vi "vibration_ysn.vi"() -> ()   [LabVIEW 2015]
uses:
  <vilib>/measure/NI_MABase.lvlib
panel:
  in  "Cluster 1":T1={"frequency"=26, "frequency 2"=8, "frequency 3"=26, " frequency 4"=26}
  out "Numeric":i32
  in  "Cluster 0":T1={"frequency"=26, "frequency 2"=8, "frequency 3"=26, " frequency 4"=26}
  in  "y 2":i32
  in  "Boolean":bool
  out "Waveform Graph":waveform(dbl)[](graph)
  in  "y":i32
  in  "Cluster":T1
  in  "Set Button":bool
  in  "appended array":waveform(dbl)[](array[waveform])
  out "x-y":u32
  in  "amplitude":dbl=2.0 format="%0.2p"
  in  "amplitude 4":dbl=2.0 format="%0.2p"
  in  "amplitude 3":dbl=2.0 format="%0.2p"
  in  "amplitude 2":dbl=2.0 format="%0.2p"
  out "frequency 4":u32=20
  out "frequency 3":u32
  in  "sampling info 4":cluster{"Fs":dbl, "#s":dbl}={"Fs"=1000.0, "#s"=250.0} {"Fs" format="%.2p"}
  in  "sampling info 3":cluster{"Fs":dbl, "#s":dbl}={"Fs"=1000.0, "#s"=250.0} {"Fs" format="%.2p"}
  in  "signal type 4":T2(ring)
  in  "signal type 3":T2(ring)
  in  "signal type 2":T2(ring)
  in  "sampling info 2":cluster{"Fs":dbl, "#s":dbl}={"Fs"=1000.0, "#s"=250.0} {"Fs" format="%.2p"}
  out "frequency 2":u32=20
  out "frequency":u32=20
  in  "signal type":T2(ring)
  in  "sampling info":cluster{"Fs":dbl, "#s":dbl}={"Fs"=1000.0, "#s"=250.0} {"Fs" format="%.2p"}
  in  "stop (F)":bool
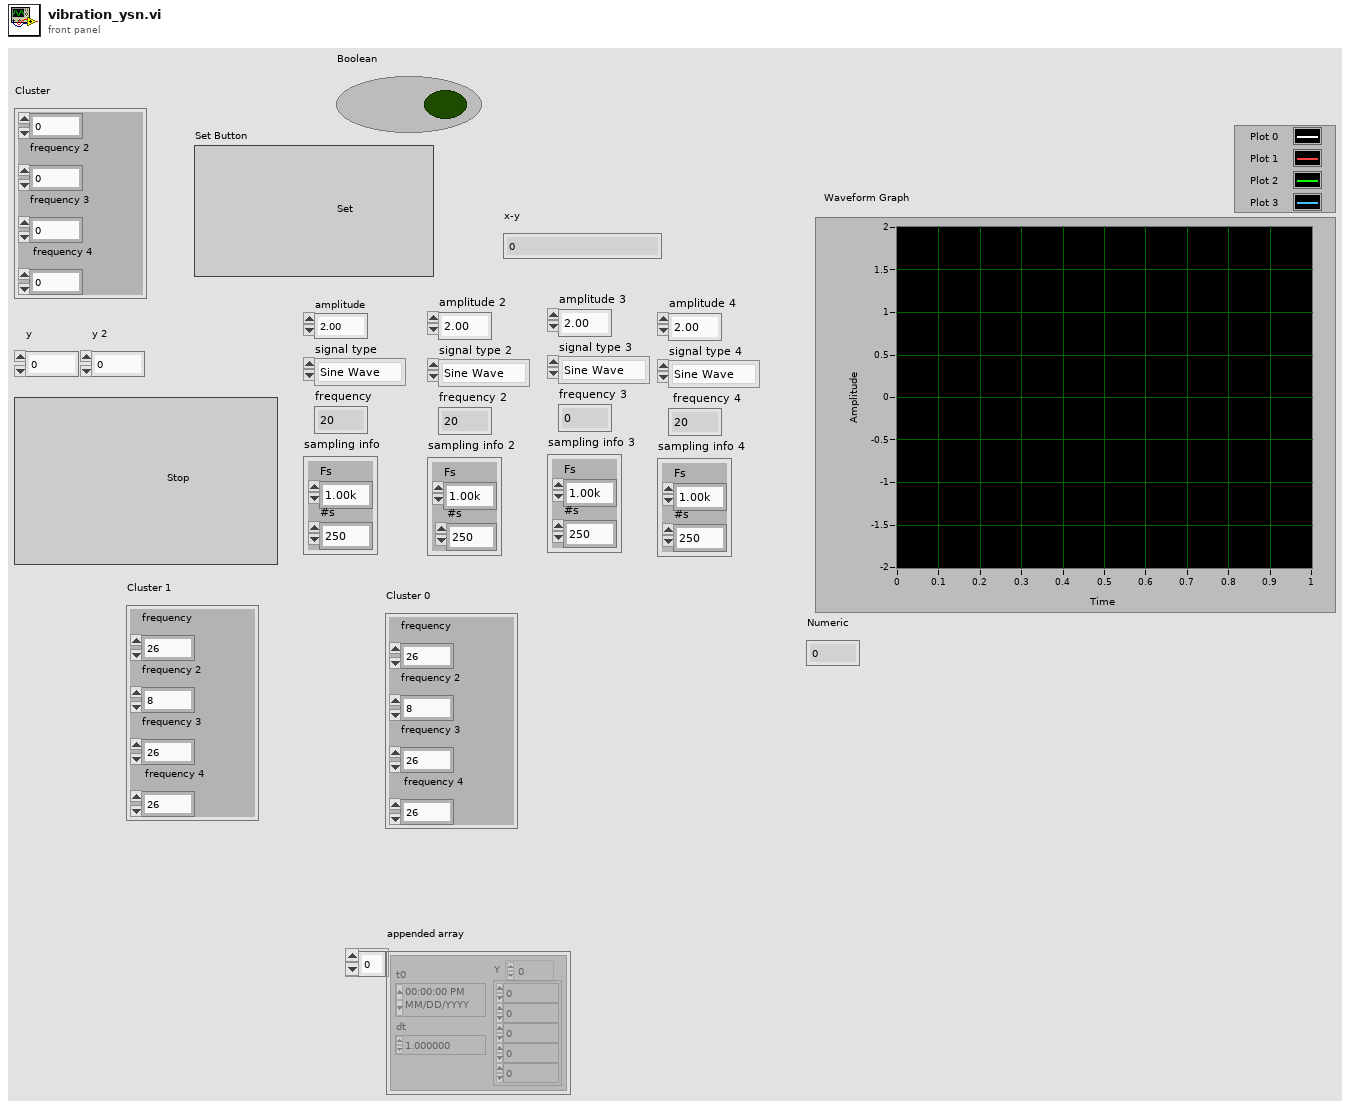
[diagram p1: front panel]
types:
  T1 = cluster{"frequency":u32, "frequency 2":u32, "frequency 3":u32, " frequency 4":u32}
  T2 = enum16{"Sine Wave", "Triangle Wave", "Square Wave", "Sawtooth Wave"}
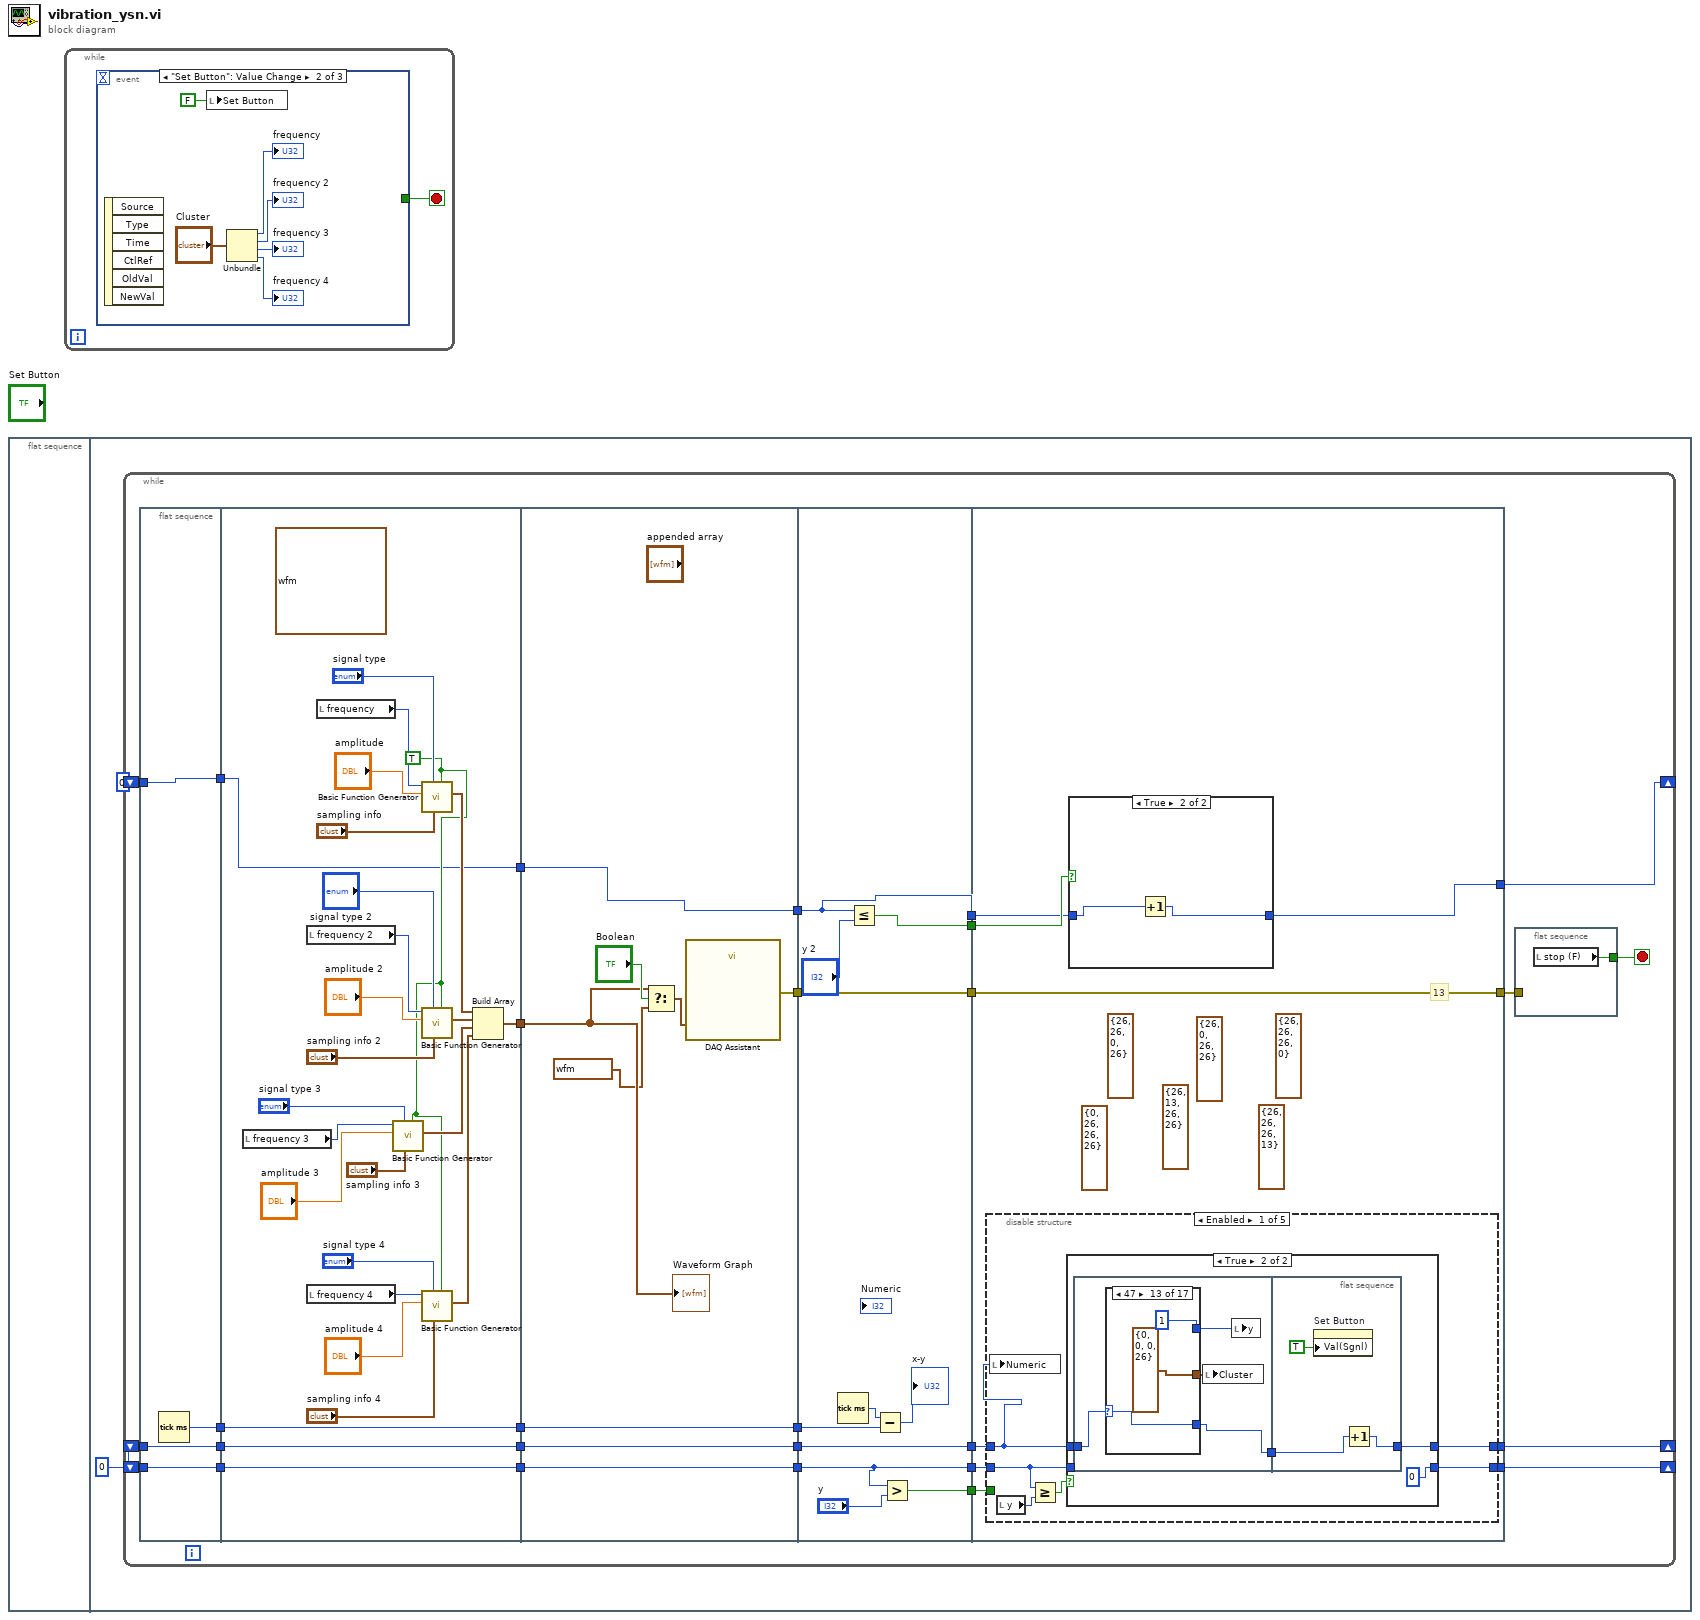
[diagram p0: block diagram]
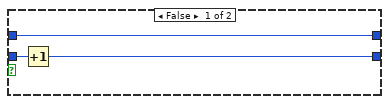
[diagram p2: hidden frame]
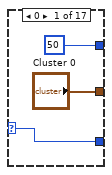
[diagram p3: hidden frame]
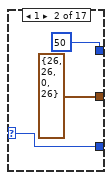
[diagram p4: hidden frame]
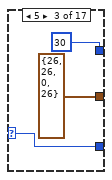
[diagram p5: hidden frame]
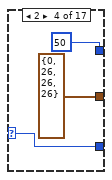
[diagram p6: hidden frame]
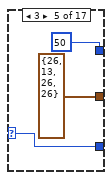
[diagram p7: hidden frame]
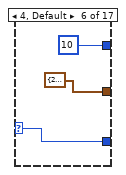
[diagram p8: hidden frame]
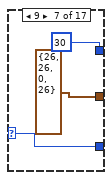
[diagram p9: hidden frame]
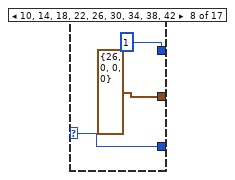
[diagram p10: hidden frame]
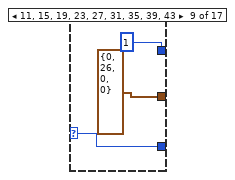
[diagram p11: hidden frame]
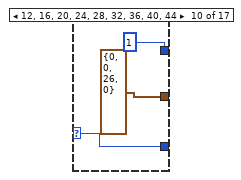
[diagram p12: hidden frame]
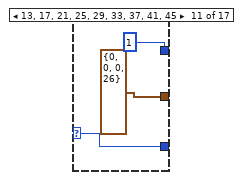
[diagram p13: hidden frame]
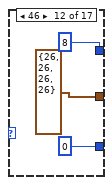
[diagram p14: hidden frame]
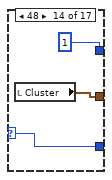
[diagram p15: hidden frame]
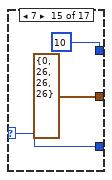
[diagram p16: hidden frame]
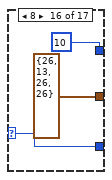
[diagram p17: hidden frame]
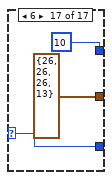
[diagram p18: hidden frame]
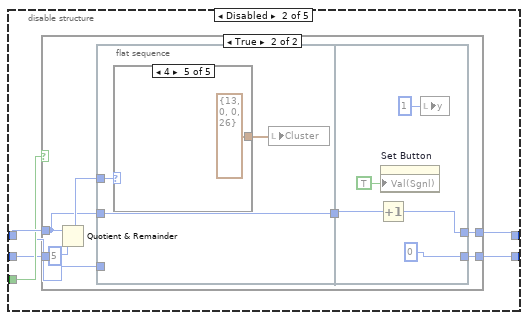
[diagram p19: hidden frame]
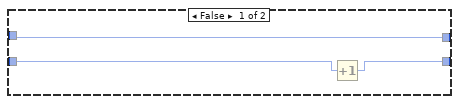
[diagram p20: hidden frame]
diagram:
  n1 = flat-sequence {
    frame #0 {
    }
    frame #1 {
      w2 = 0
      n2 = while {
        shift-right: [w19] -> _
        shift-left: w2 -> [w15]
        shift-right: [w11] -> _
        shift-left: w2 -> [w18]
        shift-right: [w6] -> _
        shift-left: 0 -> [w8]
        stop <- w30 stop-if-true
        n3 = flat-sequence {
          tunnel: [w34] -> w27
          tunnel: w18 -> [w33]
          tunnel: [w33] -> w17
          tunnel: w15 -> [w32]
          tunnel: [w32] -> w14
          tunnel: [w31] -> w9
          tunnel: w8 -> [w31]
          tunnel: [w45] -> w28
          tunnel: w27 -> [w45]
          tunnel: [w43] -> w24
          tunnel: [w37] -> w22
          tunnel: w17 -> [w38]
          tunnel: [w38] -> w16
          tunnel: w14 -> [w37]
          tunnel: [w35] -> w10
          tunnel: w9 -> [w35]
          tunnel: w28 -> [w69]
          tunnel: [w68] -> w26
          tunnel: [w69] -> w25
          tunnel: w24 -> [w63]
          tunnel: [w67] -> w23
          tunnel: w22 -> [w67]
          tunnel: w16 -> [w66]
          tunnel: [w66] -> w12
          tunnel: w10 -> [w65]
          tunnel: [w65] -> w7
          tunnel: w26 -> [w80]
          tunnel: w25 -> [w78]
          tunnel: w23 -> [w71]
          tunnel: [w80] -> w21
          tunnel: [w71] -> w20
          tunnel: [w76] -> w13
          tunnel: w12 -> [w76]
          tunnel: w7 -> [w74]
          tunnel: [w74] -> w5
          tunnel: [w73] -> w4
          tunnel: [w70] -> w3
          tunnel: [w89] -> w29
          tunnel: w21 -> [w89]
          tunnel: w20 -> [w87]
          tunnel: [w88] -> w19
          tunnel: w13 -> [w86]
          tunnel: [w85] -> w11
          tunnel: [w83] -> w6
          tunnel: w5 -> [w82]
          tunnel: w4 -> [w84]
          tunnel: w3 -> [w81]
          frame #0 {
            n4 = Tick Count (ms)() -> (millisecond timer value=w34:u32)
          }
          frame #1 {
            w36 = TRUE ("reset signal")
            (unwired) waveform(dbl) {"t0"=timestamp(0 s since 1904-01-01), "dt"=1.0, "Y"=[]} ("signal out")
            n5 = local read "frequency 3"() -> (w40:u32)
            n6 = local read "frequency 2"() -> (w41:u32)
            n7 = local read "frequency 4"() -> (w42:u32)
            n8 = local read "frequency"() -> (w39:u32)
            n9 = call <vilib>:"Basic Function Generator.vi"("reset signal"=w36, "sampling info"="sampling info 3", "signal type"="signal type 3", "amplitude"="amplitude 3", "frequency"=w40) -> ("signal out"=w51:waveform(dbl))  [unwired: 4 in, 2 out]
            n10 = call <vilib>:"Basic Function Generator.vi"("reset signal"=w36, "sampling info"="sampling info", "signal type"="signal type", "amplitude"="amplitude", "frequency"=w39) -> ("signal out"=w44:waveform(dbl))  [unwired: 4 in, 2 out]
            n11 = call <vilib>:"Basic Function Generator.vi"("reset signal"=w36, "sampling info"="sampling info 2", "signal type"="signal type 2", "amplitude"="amplitude 2", "frequency"=w41) -> ("signal out"=w57:waveform(dbl))  [unwired: 4 in, 2 out]
            n12 = call <vilib>:"Basic Function Generator.vi"("reset signal"=w36, "sampling info"="sampling info 4", "signal type"="signal type 4", "amplitude"="amplitude 4", "frequency"=w42) -> ("signal out"=w50:waveform(dbl))  [unwired: 4 in, 2 out]
            n13 = Build Array(w44, w57, w51, w50) -> (w43:waveform(dbl)[])
          }
          frame #2 {
            n14 = Select(t=w63, s="Boolean", f=waveform(dbl)[] [{"t0"=timestamp(0 s since 1904-01-01), "dt"=0.001, "Y"=[0.0, 0.0, 0.0, 0.0, 0.0, 0.0, 0.0, 0.0, 0.0, 0.0, 0.0, 0.0, 0.0, 0.0, 0.0, 0.0, 0.0, 0.0, 0.0, 0.0, 0.0, 0.0, 0.0, 0.0, 0.0, 0.0, 0.0, 0.0, 0.0, 0.0, 0.0, 0.0, 0.0, 0.0, 0.0, 0.0, 0.0, 0.0, 0.0, 0.0, 0.0, 0.0, 0.0, 0.0, 0.0, 0.0, 0.0, 0.0, 0.0, 0.0, 0.0, 0.0, 0.0, 0.0, 0.0, 0.0, 0.0, 0.0, 0.0, 0.0, 0.0, 0.0, 0.0, 0.0, 0.0, 0.0, 0.0, 0.0, 0.0, 0.0, 0.0, 0.0, 0.0, 0.0, 0.0, 0.0, 0.0, 0.0, 0.0, 0.0, 0.0, 0.0, 0.0, 0.0, 0.0, 0.0, 0.0, 0.0, 0.0, 0.0, 0.0, 0.0, 0.0, 0.0, 0.0, 0.0, 0.0, 0.0, 0.0, 0.0, 0.0, 0.0, 0.0, 0.0, 0.0, 0.0, 0.0, 0.0, 0.0, 0.0, 0.0, 0.0, 0.0, 0.0, 0.0, 0.0, 0.0, 0.0, 0.0, 0.0, 0.0, 0.0, 0.0, 0.0, 0.0, 0.0, 0.0, 0.0, 0.0, 0.0, 0.0, 0.0, 0.0, 0.0, 0.0, 0.0, 0.0, 0.0, 0.0, 0.0, 0.0, 0.0, 0.0, 0.0, 0.0, 0.0, 0.0, 0.0, 0.0, 0.0, 0.0, 0.0, 0.0, 0.0, 0.0, 0.0, 0.0, 0.0, 0.0, 0.0, 0.0, 0.0, 0.0, 0.0, 0.0, 0.0, 0.0, 0.0, 0.0, 0.0, 0.0, 0.0, 0.0, 0.0, 0.0, 0.0, 0.0, 0.0, 0.0, 0.0, 0.0, 0.0, 0.0, 0.0, 0.0, 0.0, 0.0, 0.0, 0.0, 0.0, 0.0, 0.0, 0.0, 0.0, 0.0, 0.0, 0.0, 0.0, 0.0, 0.0, 0.0, 0.0, 0.0, 0.0, 0.0, 0.0, 0.0, 0.0, 0.0, 0.0, 0.0, 0.0, 0.0, 0.0, 0.0, 0.0, 0.0, 0.0, 0.0, 0.0, 0.0, 0.0, 0.0, 0.0, 0.0, 0.0, 0.0, 0.0, 0.0, 0.0, 0.0, 0.0, 0.0, 0.0, 0.0, 0.0, 0.0, 0.0, 0.0, 0.0, 0.0, 0.0, 0.0, 0.0, 0.0, 0.0, 0.0, 0.0, 0.0, 0.0]}, {"t0"=timestamp(0 s since 1904-01-01), "dt"=0.001, "Y"=[0.0, 0.0, 0.0, 0.0, 0.0, 0.0, 0.0, 0.0, 0.0, 0.0, 0.0, 0.0, 0.0, 0.0, 0.0, 0.0, 0.0, 0.0, 0.0, 0.0, 0.0, 0.0, 0.0, 0.0, 0.0, 0.0, 0.0, 0.0, 0.0, 0.0, 0.0, 0.0, 0.0, 0.0, 0.0, 0.0, 0.0, 0.0, 0.0, 0.0, 0.0, 0.0, 0.0, 0.0, 0.0, 0.0, 0.0, 0.0, 0.0, 0.0, 0.0, 0.0, 0.0, 0.0, 0.0, 0.0, 0.0, 0.0, 0.0, 0.0, 0.0, 0.0, 0.0, 0.0, 0.0, 0.0, 0.0, 0.0, 0.0, 0.0, 0.0, 0.0, 0.0, 0.0, 0.0, 0.0, 0.0, 0.0, 0.0, 0.0, 0.0, 0.0, 0.0, 0.0, 0.0, 0.0, 0.0, 0.0, 0.0, 0.0, 0.0, 0.0, 0.0, 0.0, 0.0, 0.0, 0.0, 0.0, 0.0, 0.0, 0.0, 0.0, 0.0, 0.0, 0.0, 0.0, 0.0, 0.0, 0.0, 0.0, 0.0, 0.0, 0.0, 0.0, 0.0, 0.0, 0.0, 0.0, 0.0, 0.0, 0.0, 0.0, 0.0, 0.0, 0.0, 0.0, 0.0, 0.0, 0.0, 0.0, 0.0, 0.0, 0.0, 0.0, 0.0, 0.0, 0.0, 0.0, 0.0, 0.0, 0.0, 0.0, 0.0, 0.0, 0.0, 0.0, 0.0, 0.0, 0.0, 0.0, 0.0, 0.0, 0.0, 0.0, 0.0, 0.0, 0.0, 0.0, 0.0, 0.0, 0.0, 0.0, 0.0, 0.0, 0.0, 0.0, 0.0, 0.0, 0.0, 0.0, 0.0, 0.0, 0.0, 0.0, 0.0, 0.0, 0.0, 0.0, 0.0, 0.0, 0.0, 0.0, 0.0, 0.0, 0.0, 0.0, 0.0, 0.0, 0.0, 0.0, 0.0, 0.0, 0.0, 0.0, 0.0, 0.0, 0.0, 0.0, 0.0, 0.0, 0.0, 0.0, 0.0, 0.0, 0.0, 0.0, 0.0, 0.0, 0.0, 0.0, 0.0, 0.0, 0.0, 0.0, 0.0, 0.0, 0.0, 0.0, 0.0, 0.0, 0.0, 0.0, 0.0, 0.0, 0.0, 0.0, 0.0, 0.0, 0.0, 0.0, 0.0, 0.0, 0.0, 0.0, 0.0, 0.0, 0.0, 0.0, 0.0, 0.0, 0.0, 0.0, 0.0, 0.0, 0.0, 0.0, 0.0, 0.0, 0.0, 0.0]}, {"t0"=timestamp(0 s since 1904-01-01), "dt"=0.001, "Y"=[0.0, 0.0, 0.0, 0.0, 0.0, 0.0, 0.0, 0.0, 0.0, 0.0, 0.0, 0.0, 0.0, 0.0, 0.0, 0.0, 0.0, 0.0, 0.0, 0.0, 0.0, 0.0, 0.0, 0.0, 0.0, 0.0, 0.0, 0.0, 0.0, 0.0, 0.0, 0.0, 0.0, 0.0, 0.0, 0.0, 0.0, 0.0, 0.0, 0.0, 0.0, 0.0, 0.0, 0.0, 0.0, 0.0, 0.0, 0.0, 0.0, 0.0, 0.0, 0.0, 0.0, 0.0, 0.0, 0.0, 0.0, 0.0, 0.0, 0.0, 0.0, 0.0, 0.0, 0.0, 0.0, 0.0, 0.0, 0.0, 0.0, 0.0, 0.0, 0.0, 0.0, 0.0, 0.0, 0.0, 0.0, 0.0, 0.0, 0.0, 0.0, 0.0, 0.0, 0.0, 0.0, 0.0, 0.0, 0.0, 0.0, 0.0, 0.0, 0.0, 0.0, 0.0, 0.0, 0.0, 0.0, 0.0, 0.0, 0.0, 0.0, 0.0, 0.0, 0.0, 0.0, 0.0, 0.0, 0.0, 0.0, 0.0, 0.0, 0.0, 0.0, 0.0, 0.0, 0.0, 0.0, 0.0, 0.0, 0.0, 0.0, 0.0, 0.0, 0.0, 0.0, 0.0, 0.0, 0.0, 0.0, 0.0, 0.0, 0.0, 0.0, 0.0, 0.0, 0.0, 0.0, 0.0, 0.0, 0.0, 0.0, 0.0, 0.0, 0.0, 0.0, 0.0, 0.0, 0.0, 0.0, 0.0, 0.0, 0.0, 0.0, 0.0, 0.0, 0.0, 0.0, 0.0, 0.0, 0.0, 0.0, 0.0, 0.0, 0.0, 0.0, 0.0, 0.0, 0.0, 0.0, 0.0, 0.0, 0.0, 0.0, 0.0, 0.0, 0.0, 0.0, 0.0, 0.0, 0.0, 0.0, 0.0, 0.0, 0.0, 0.0, 0.0, 0.0, 0.0, 0.0, 0.0, 0.0, 0.0, 0.0, 0.0, 0.0, 0.0, 0.0, 0.0, 0.0, 0.0, 0.0, 0.0, 0.0, 0.0, 0.0, 0.0, 0.0, 0.0, 0.0, 0.0, 0.0, 0.0, 0.0, 0.0, 0.0, 0.0, 0.0, 0.0, 0.0, 0.0, 0.0, 0.0, 0.0, 0.0, 0.0, 0.0, 0.0, 0.0, 0.0, 0.0, 0.0, 0.0, 0.0, 0.0, 0.0, 0.0, 0.0, 0.0, 0.0, 0.0, 0.0, 0.0, 0.0, 0.0, 0.0, 0.0, 0.0, 0.0, 0.0, 0.0]}, {"t0"=timestamp(0 s since 1904-01-01), "dt"=0.001, "Y"=[0.0, 0.0, 0.0, 0.0, 0.0, 0.0, 0.0, 0.0, 0.0, 0.0, 0.0, 0.0, 0.0, 0.0, 0.0, 0.0, 0.0, 0.0, 0.0, 0.0, 0.0, 0.0, 0.0, 0.0, 0.0, 0.0, 0.0, 0.0, 0.0, 0.0, 0.0, 0.0, 0.0, 0.0, 0.0, 0.0, 0.0, 0.0, 0.0, 0.0, 0.0, 0.0, 0.0, 0.0, 0.0, 0.0, 0.0, 0.0, 0.0, 0.0, 0.0, 0.0, 0.0, 0.0, 0.0, 0.0, 0.0, 0.0, 0.0, 0.0, 0.0, 0.0, 0.0, 0.0, 0.0, 0.0, 0.0, 0.0, 0.0, 0.0, 0.0, 0.0, 0.0, 0.0, 0.0, 0.0, 0.0, 0.0, 0.0, 0.0, 0.0, 0.0, 0.0, 0.0, 0.0, 0.0, 0.0, 0.0, 0.0, 0.0, 0.0, 0.0, 0.0, 0.0, 0.0, 0.0, 0.0, 0.0, 0.0, 0.0, 0.0, 0.0, 0.0, 0.0, 0.0, 0.0, 0.0, 0.0, 0.0, 0.0, 0.0, 0.0, 0.0, 0.0, 0.0, 0.0, 0.0, 0.0, 0.0, 0.0, 0.0, 0.0, 0.0, 0.0, 0.0, 0.0, 0.0, 0.0, 0.0, 0.0, 0.0, 0.0, 0.0, 0.0, 0.0, 0.0, 0.0, 0.0, 0.0, 0.0, 0.0, 0.0, 0.0, 0.0, 0.0, 0.0, 0.0, 0.0, 0.0, 0.0, 0.0, 0.0, 0.0, 0.0, 0.0, 0.0, 0.0, 0.0, 0.0, 0.0, 0.0, 0.0, 0.0, 0.0, 0.0, 0.0, 0.0, 0.0, 0.0, 0.0, 0.0, 0.0, 0.0, 0.0, 0.0, 0.0, 0.0, 0.0, 0.0, 0.0, 0.0, 0.0, 0.0, 0.0, 0.0, 0.0, 0.0, 0.0, 0.0, 0.0, 0.0, 0.0, 0.0, 0.0, 0.0, 0.0, 0.0, 0.0, 0.0, 0.0, 0.0, 0.0, 0.0, 0.0, 0.0, 0.0, 0.0, 0.0, 0.0, 0.0, 0.0, 0.0, 0.0, 0.0, 0.0, 0.0, 0.0, 0.0, 0.0, 0.0, 0.0, 0.0, 0.0, 0.0, 0.0, 0.0, 0.0, 0.0, 0.0, 0.0, 0.0, 0.0, 0.0, 0.0, 0.0, 0.0, 0.0, 0.0, 0.0, 0.0, 0.0, 0.0, 0.0, 0.0, 0.0, 0.0, 0.0, 0.0, 0.0, 0.0]}]) -> (s? t:f=w62:waveform(dbl)[])
            n15 = call "DAQ Assistant"("data"=w62) -> ("error out"=w68:errorcluster)  [unwired: 17 in, 1 out]
            "Waveform Graph" <- w63
          }
          frame #3 {
            n16 = Tick Count (ms)() -> (millisecond timer value=w79:u32)
            n17 = Less Or Equal?(x=w74, y="y 2") -> (x <= y?=w73:bool)
            n18 = Subtract(x=w79, y=w78) -> (x-y=→"x-y":u32)
            n19 = Greater?(x=w71, y="y") -> (0:w70:bool)
          }
          frame #4 {
            (unwired) T1 {"frequency"=26, "frequency 2"=26, "frequency 3"=26, " frequency 4"=13} ("Cluster 8")
            (unwired) T1 {"frequency"=26, "frequency 2"=13, "frequency 3"=26, " frequency 4"=26} ("Cluster 7")
            (unwired) T1 {"frequency"=0, "frequency 2"=26, "frequency 3"=26, " frequency 4"=26} ("Cluster 6")
            (unwired) T1 {"frequency"=26, "frequency 2"=26, "frequency 3"=26, " frequency 4"=0} ("Cluster")
            (unwired) T1 {"frequency"=26, "frequency 2"=0, "frequency 3"=26, " frequency 4"=26} ("Cluster")
            (unwired) T1 {"frequency"=26, "frequency 2"=26, "frequency 3"=0, " frequency 4"=26} ("Cluster")
            # "13"
            n20 = disable-structure shown="Enabled" {
              disable-tunnel: [w95 w163 _ w193 w261] -> w88
              disable-tunnel: w87 -> [w94 w161 _ w192 w260]
              disable-tunnel: w86 -> [w91 w165 _ w189 w256]
              disable-tunnel: [w93 w164 _ w191 w259] -> w85
              disable-tunnel: w81 -> [_ w162 _ _ _]
              frame Enabled {
                n21 = local write "Numeric"(w91) -> ()
                n22 = local read "y"() -> (w90:i32)
                n23 = Greater Or Equal?(x=w94, y=w90) -> (x >= y?=w92:bool)
                n24 = case shown="True" w92 {
                  tunnel: [w97 0] -> w95
                  tunnel: w94 -> [w98 _]
                  tunnel: w91 -> [w96 w101]
                  tunnel: [w96 w100] -> w93
                  frame False {
                    n25 = Increment(x=w98) -> (x+1=w97:i32)
                  }
                  frame True {
                    n26 = flat-sequence {
                      tunnel: w101 -> [w103]
                      tunnel: [w105] -> w99
                      tunnel: [w160] -> w100
                      tunnel: w99 -> [w159]
                      frame #0 {
                        n27 = case shown="47" w103 {
                          selector: w103 -> [w108 w111 w114 w117 w120 w123 w125 w128 w131 w134 w137 _ w143 w147 w150 w153 w155]
                          tunnel: ["Cluster 0" T1 {"frequency"=26, "frequency 2"=26, "frequency 3"=0, " frequency 4"=26} ("Cluster 1") T1 {"frequency"=26, "frequency 2"=26, "frequency 3"=0, " frequency 4"=26} ("Cluster 1") T1 {"frequency"=0, "frequency 2"=26, "frequency 3"=26, " frequency 4"=26} ("Cluster 2") T1 {"frequency"=26, "frequency 2"=13, "frequency 3"=26, " frequency 4"=26} ("Cluster 3") T1 {"frequency"=26, "frequency 2"=26, "frequency 3"=26, " frequency 4"=13} ("Cluster 4") T1 {"frequency"=26, "frequency 2"=26, "frequency 3"=0, " frequency 4"=26} ("Cluster 5") T1 {"frequency"=26, "frequency 2"=0, "frequency 3"=0, " frequency 4"=0} ("Cluster 5") T1 {"frequency"=0, "frequency 2"=26, "frequency 3"=0, " frequency 4"=0} ("Cluster 5") T1 {"frequency"=0, "frequency 2"=0, "frequency 3"=26, " frequency 4"=0} ("Cluster 5") T1 {"frequency"=0, "frequency 2"=0, "frequency 3"=0, " frequency 4"=26} ("Cluster 5") T1 {"frequency"=26, "frequency 2"=26, "frequency 3"=26, " frequency 4"=26} ("Cluster 5") T1 {"frequency"=0, "frequency 2"=0, "frequency 3"=0, " frequency 4"=26} ("Cluster 5") w146 T1 {"frequency"=0, "frequency 2"=26, "frequency 3"=26, " frequency 4"=26} ("Cluster 6") T1 {"frequency"=26, "frequency 2"=13, "frequency 3"=26, " frequency 4"=26} ("Cluster 6") T1 {"frequency"=26, "frequency 2"=26, "frequency 3"=26, " frequency 4"=13} ("Cluster 6")] -> w106
                          tunnel: [w108 w111 w114 w117 w120 w123 w125 w128 w131 w134 w137 0 w143 w147 w150 w153 w155] -> w105
                          tunnel: [50 ("y") 50 ("y") 30 ("y") 50 ("y") 50 ("y") 10 ("y") 30 ("y") 1 ("y") 1 ("y") 1 ("y") 1 ("y") 8 ("y") 1 ("y") 1 ("y") 10 ("y") 10 ("y") 10 ("y")] -> w104
                          frame 0 {
                          }
                          frame 1 {
                          }
                          frame 5 {
                          }
                          frame 2 {
                          }
                          frame 3 {
                          }
                          frame 4, Default {
                          }
                          frame 9 {
                          }
                          frame 10, 14, 18, 22, 26, 30, 34, 38, 42 {
                          }
                          frame 11, 15, 19, 23, 27, 31, 35, 39, 43 {
                          }
                          frame 12, 16, 20, 24, 28, 32, 36, 40, 44 {
                          }
                          frame 13, 17, 21, 25, 29, 33, 37, 41, 45 {
                          }
                          frame 46 {
                          }
                          frame 47 {
                          }
                          frame 48 {
                            n28 = local read "Cluster"() -> (w146:T1)
                          }
                          frame 7 {
                          }
                          frame 8 {
                          }
                          frame 6 {
                          }
                        }
                        n29 = local write "Cluster"(w106) -> ()
                        n30 = local write "y"(w104) -> ()
                      }
                      frame #1 {
                        n31 = property on="Set Button" class="Bool (strict)"("Val(Sgnl)"=TRUE ("Value (Signaling)")) -> ()  [unwired: 2 in, 2 out]
                        n32 = Increment(x=w159) -> (x+1=w160:i32)
                      }
                    }
                  }
                }
              }
              frame Disabled {
                n33 = case shown="True" w162 {
                  tunnel: w165 -> [w166 w169]
                  tunnel: [w166 w172] -> w164
                  tunnel: [w167 w171] -> w163
                  tunnel: w161 -> [w168 _]
                  frame False {
                    n34 = Increment(x=w168) -> (x+1=w167:i32)
                  }
                  frame True {
                    n35 = Quotient & Remainder(x=w169, y=5) -> (x-y*floor(x/y)=w173:i32)  [unwired: 1 out]
                    n36 = flat-sequence {
                      tunnel: w173 -> [w177]
                      tunnel: w169 -> [_]
                      tunnel: [w175] -> w170
                      tunnel: w169 -> [w175]
                      tunnel: [w184] -> w172
                      tunnel: [0] -> w171
                      tunnel: w170 -> [w185]
                      frame #0 {
                        n37 = case shown="4" w177 {
                          tunnel: [T1 {"frequency"=26, "frequency 2"=26, "frequency 3"=26, " frequency 4"=26} ("Cluster 6") T1 {"frequency"=26, "frequency 2"=13, "frequency 3"=0, " frequency 4"=0} ("Cluster 6") T1 {"frequency"=0, "frequency 2"=26, "frequency 3"=13, " frequency 4"=0} ("Cluster 6") T1 {"frequency"=0, "frequency 2"=0, "frequency 3"=26, " frequency 4"=13} ("Cluster 6") T1 {"frequency"=13, "frequency 2"=0, "frequency 3"=0, " frequency 4"=26} ("Cluster 6")] -> w176
                          frame 0, Default {
                          }
                          frame 1 {
                          }
                          frame 3 {
                          }
                          frame 2 {
                          }
                          frame 4 {
                          }
                        }
                        n38 = local write "Cluster"(w176) -> ()
                      }
                      frame #1 {
                        n39 = Increment(x=w185) -> (x+1=w184:i32)
                        n40 = property on="Set Button" class="Bool (strict)"("Val(Sgnl)"=TRUE ("Value (Signaling)")) -> ()  [unwired: 2 in, 2 out]
                        n41 = local write "y"(1 ("y")) -> ()
                      }
                    }
                  }
                }
              }
              frame Disabled {
              }
              frame Disabled {
                n42 = local write "Numeric"(w189) -> ()
                n43 = local read "y"() -> (w188:i32)
                n44 = Greater Or Equal?(x=w192, y=w188) -> (x >= y?=w190:bool)
                n45 = case shown="True" w190 {
                  tunnel: [w195 0] -> w193
                  tunnel: w192 -> [w196 _]
                  tunnel: w189 -> [w194 w199]
                  tunnel: [w194 w198] -> w191
                  frame False {
                    n46 = Increment(x=w196) -> (x+1=w195:i32)
                  }
                  frame True {
                    n47 = flat-sequence {
                      tunnel: w199 -> [w203]
                      tunnel: [w202] -> w197
                      tunnel: [w254] -> w198
                      tunnel: w197 -> [w253]
                      frame #0 {
                        n48 = case shown="10, 14, 18, 22, 26, 30, 34, 38, 42" w203 {
                          selector: w203 -> [w206 w209 w212 w215 w218 w221 w223 w226 w229 w232 w235 _ w241 w245 w248 w250]
                          tunnel: ["Cluster 1" T1 {"frequency"=26, "frequency 2"=26, "frequency 3"=0, " frequency 4"=26} ("Cluster 1") T1 {"frequency"=26, "frequency 2"=26, "frequency 3"=0, " frequency 4"=26} ("Cluster 1") T1 {"frequency"=0, "frequency 2"=26, "frequency 3"=26, " frequency 4"=26} ("Cluster 2") T1 {"frequency"=26, "frequency 2"=13, "frequency 3"=26, " frequency 4"=26} ("Cluster 3") T1 {"frequency"=26, "frequency 2"=26, "frequency 3"=26, " frequency 4"=13} ("Cluster 4") T1 {"frequency"=26, "frequency 2"=26, "frequency 3"=0, " frequency 4"=26} ("Cluster 5") T1 {"frequency"=26, "frequency 2"=0, "frequency 3"=0, " frequency 4"=0} ("Cluster 5") T1 {"frequency"=0, "frequency 2"=26, "frequency 3"=0, " frequency 4"=0} ("Cluster 5") T1 {"frequency"=0, "frequency 2"=0, "frequency 3"=26, " frequency 4"=0} ("Cluster 5") T1 {"frequency"=0, "frequency 2"=0, "frequency 3"=0, " frequency 4"=26} ("Cluster 5") T1 {"frequency"=26, "frequency 2"=26, "frequency 3"=26, " frequency 4"=26} ("Cluster 5") T1 {"frequency"=0, "frequency 2"=0, "frequency 3"=0, " frequency 4"=26} ("Cluster 5") T1 {"frequency"=0, "frequency 2"=26, "frequency 3"=26, " frequency 4"=26} ("Cluster 6") T1 {"frequency"=26, "frequency 2"=13, "frequency 3"=26, " frequency 4"=26} ("Cluster 6") T1 {"frequency"=26, "frequency 2"=26, "frequency 3"=26, " frequency 4"=13} ("Cluster 6")] -> w204
                          tunnel: [w206 w209 w212 w215 w218 w221 w223 w226 w229 w232 w235 0 w241 w245 w248 w250] -> w202
                          tunnel: [50 ("y") 50 ("y") 30 ("y") 50 ("y") 50 ("y") 10 ("y") 30 ("y") 1 ("y") 1 ("y") 1 ("y") 1 ("y") 8 ("y") 1 ("y") 10 ("y") 10 ("y") 10 ("y")] -> w201
                          frame 0 {
                          }
                          frame 1 {
                          }
                          frame 5 {
                          }
                          frame 2 {
                          }
                          frame 3 {
                          }
                          frame 4, Default {
                          }
                          frame 9 {
                          }
                          frame 10, 14, 18, 22, 26, 30, 34, 38, 42 {
                          }
                          frame 11, 15, 19, 23, 27, 31, 35, 39, 43 {
                          }
                          frame 12, 16, 20, 24, 28, 32, 36, 40, 44 {
                          }
                          frame 13, 17, 21, 25, 29, 33, 37, 41, 45 {
                          }
                          frame 46 {
                          }
                          frame 47 {
                          }
                          frame 7 {
                          }
                          frame 8 {
                          }
                          frame 6 {
                          }
                        }
                        n49 = local write "Cluster"(w204) -> ()
                        n50 = local write "y"(w201) -> ()
                      }
                      frame #1 {
                        n51 = property on="Set Button" class="Bool (strict)"("Val(Sgnl)"=TRUE ("Value (Signaling)")) -> ()  [unwired: 2 in, 2 out]
                        n52 = Increment(x=w253) -> (x+1=w254:i32)
                      }
                    }
                  }
                }
              }
              frame Disabled {
                n53 = local read "y"() -> (w257:i32)
                n54 = local write "Numeric"(w256) -> ()
                n55 = Greater Or Equal?(x=w260, y=w257) -> (x >= y?=w258:bool)
                n56 = case shown="True" w258 {
                  tunnel: [w263 0] -> w261
                  tunnel: w260 -> [w264 _]
                  tunnel: w256 -> [w262 w267]
                  tunnel: [w262 w266] -> w259
                  frame False {
                    n57 = Increment(x=w264) -> (x+1=w263:i32)
                  }
                  frame True {
                    n58 = flat-sequence {
                      tunnel: w267 -> [w271]
                      tunnel: [w270] -> w265
                      tunnel: [w304] -> w266
                      tunnel: w265 -> [w303]
                      frame #0 {
                        n59 = case shown="0" w271 {
                          selector: w271 -> [w274 w277 w280 w283 w286 w289 _ w295 w298 w300]
                          tunnel: [w275 T1 {"frequency"=26, "frequency 2"=26, "frequency 3"=0, " frequency 4"=26} ("Cluster 1") T1 {"frequency"=26, "frequency 2"=26, "frequency 3"=0, " frequency 4"=26} ("Cluster 1") T1 {"frequency"=0, "frequency 2"=26, "frequency 3"=26, " frequency 4"=26} ("Cluster 2") T1 {"frequency"=26, "frequency 2"=13, "frequency 3"=26, " frequency 4"=26} ("Cluster 3") T1 {"frequency"=26, "frequency 2"=26, "frequency 3"=26, " frequency 4"=13} ("Cluster 4") T1 {"frequency"=26, "frequency 2"=26, "frequency 3"=0, " frequency 4"=26} ("Cluster 5") T1 {"frequency"=0, "frequency 2"=26, "frequency 3"=26, " frequency 4"=26} ("Cluster 6") T1 {"frequency"=26, "frequency 2"=13, "frequency 3"=26, " frequency 4"=26} ("Cluster 6") T1 {"frequency"=26, "frequency 2"=26, "frequency 3"=26, " frequency 4"=13} ("Cluster 6")] -> w272
                          tunnel: [w274 w277 w280 w283 w286 w289 0 w295 w298 w300] -> w270
                          tunnel: [50 ("y") 50 ("y") 30 ("y") 50 ("y") 50 ("y") 10 ("y") 10 ("y") 10 ("y") 10 ("y") 10 ("y")] -> w269
                          frame 0 {
                          }
                          frame 1 {
                          }
                          frame 5 {
                          }
                          frame 2 {
                          }
                          frame 3 {
                          }
                          frame 4, Default {
                          }
                          frame 9 {
                          }
                          frame 7 {
                          }
                          frame 8 {
                          }
                          frame 6 {
                          }
                        }
                        n60 = local write "Cluster"(w272) -> ()
                        n61 = local write "y"(w269) -> ()
                      }
                      frame #1 {
                        n62 = property on="Set Button" class="Bool (strict)"("Val(Sgnl)"=TRUE ("Value (Signaling)")) -> ()  [unwired: 2 in, 2 out]
                        n63 = Increment(x=w303) -> (x+1=w304:i32)
                      }
                    }
                  }
                }
              }
            }
            n64 = case shown="True" w84 {
              tunnel: [0 w307] -> w83
              tunnel: w82 -> [_ w308]
              frame False {
              }
              frame True {
                n65 = Increment(x=w308) -> (x+1=w307:i32)
              }
            }
          }
        }
        n66 = flat-sequence {
          tunnel: w29 -> [_]
          tunnel: [w309] -> w30
          frame #0 {
            n67 = local read "stop (F)"() -> (w309:bool)
          }
        }
      }
    }
  }
  n68 = while {
    stop <- w310 stop-if-true
    n69 = event shown="[1] \"Set Button\": Value Change" {
      selector: _ -> [_ _ _]
      dyn-events: _ -> [_ _ _]
      timeout: _ -> [_ _ _]
      tunnel: [_ _ "stop (F)"] -> w310
      event Timeout {
        n70 = event-data() -> ()  [unwired: 1 in, 3 out]
      }
      event "Set Button": Value Change {
        n71 = event-data() -> ()  [unwired: 1 in, 6 out]
        n72 = local write "Set Button"(FALSE ("Set Button")) -> ()
        n73 = Unbundle("Cluster") -> ("frequency"=→"frequency":u32, "frequency 2"=→"frequency 2":u32, "frequency 3"=→"frequency 3":u32, "frequency 4"=→"frequency 4":u32)
      }
      event "stop (F)": Value Change {
        n74 = event-data() -> ()  [unwired: 1 in, 6 out]
      }
    }
  }
